vi "Get Serial Number.vi"(8 "error in":errorcluster, 11 "PPT in":refnum<class "PPT.lvclass">) -> (0 "error out":errorcluster, 2 "SN":string, 3 "PPT out":refnum<class "PPT.lvclass">)   [LabVIEW 2014, in "PPT Library.lvlib" / "PPT.lvclass"]
doc: "Set the transceiver operating parameters. See PPT documentation to determine how the input parameter is applied."
uses:
  PPT.lvclass
  reusable/Session APIs/Serial/Serial Session.lvclass
  PPT.lvclass/PPT.ctl
  Configurable Device/Configurable Device.lvclass/Configurable Device.ctl
  Configurable Device/Accessors/Write SN.vi
  reusable/Session APIs/Serial/Public/Asynchronous Write.vi
  reusable/Session APIs/Serial/Public/Asynchronous Read.vi
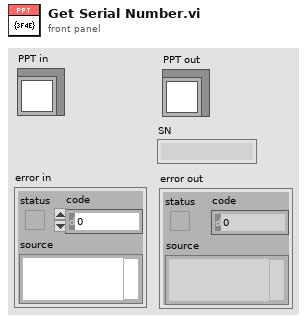
[diagram p1: front panel]
types:
  T1 = typedef "Session - Root.lvclass/Session Handle.ctl" = refnum<data-value>
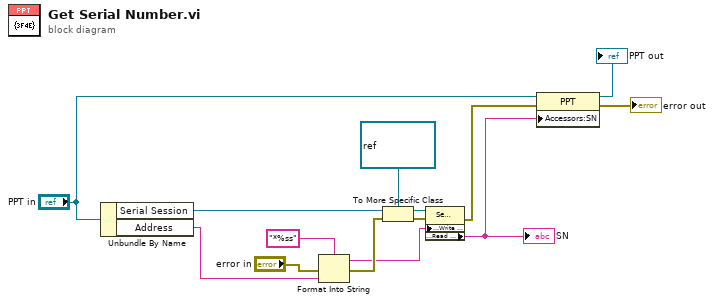
[diagram p0: block diagram]
diagram:
  n1 = Unbundle By Name("PPT in") -> ("Serial Session"=w7:T1, "Address"=w8:string)
  n2 = Format Into String(format string="*%ss", error in="error in", w8) -> (resulting string=w9:string, error out=w10:errorcluster)  [unwired: 1 in]
  n3 = To More Specific Class(target class=refnum<data-value> refnum ("Serial Session"), reference=w7, error in=w10) -> (specific class reference=w13:refnum<data-value>, error out=w12:errorcluster)
  n4 = property class="Serial Session"(reference=w13, error in=w12, "Public:Write - Asynchronous"=w9) -> (error out=w2:errorcluster, "Public:Read - Asynchronous"=w4:string)  [unwired: 1 out]
  "SN" <- w4
  n5 = property class="PPT"(reference="PPT in", error in=w2, "Accessors:SN"=w4) -> (reference out=→"PPT out":refnum<class "PPT.lvclass">, error out=→"error out":errorcluster)
